vi "Read XML HW Configuration File_Parse Channels.vi"(8 "error in (no error)":errorcluster, 11 "channel1553":refnum<k24>[](array[refnum])) -> (0 "error out":errorcluster, 2 "channels":T1[](array[typedef]))   [LabVIEW 2017, in "Ballard 1553 System Explorer.lvlib"]
doc: "This VI parses the XML HW DB."
uses:
  Ballard 1553 System Explorer.lvlib
  Ballard_Channel.ctl
  Ballard_BC.ctl
  Ballard_message.ctl
  Ballard_messageType.ctl
  Ballard_CWD1.ctl
  Ballard_CWD2.ctl
  Ballard_minorFrame.ctl
  Ballard_majorFrame.ctl
  Ballard_acyclicFrame.ctl
  Ballard_RT.ctl
  Ballard_RT subAddress.ctl
  Ballard_RT direction.ctl
  Ballard_RT rtMode.ctl
  Ballard_RT modeCode.ctl
  D:/Ballard-1553-Custom-Device Inline Async/Source/System Explorer/SubVIs/Parse XML Ballard/Ballard_BTI_XML_MIL_STD_1553_Deserializer.dll
  Ballard_BTI_XML_MIL_STD_1553_Deserializer.dll
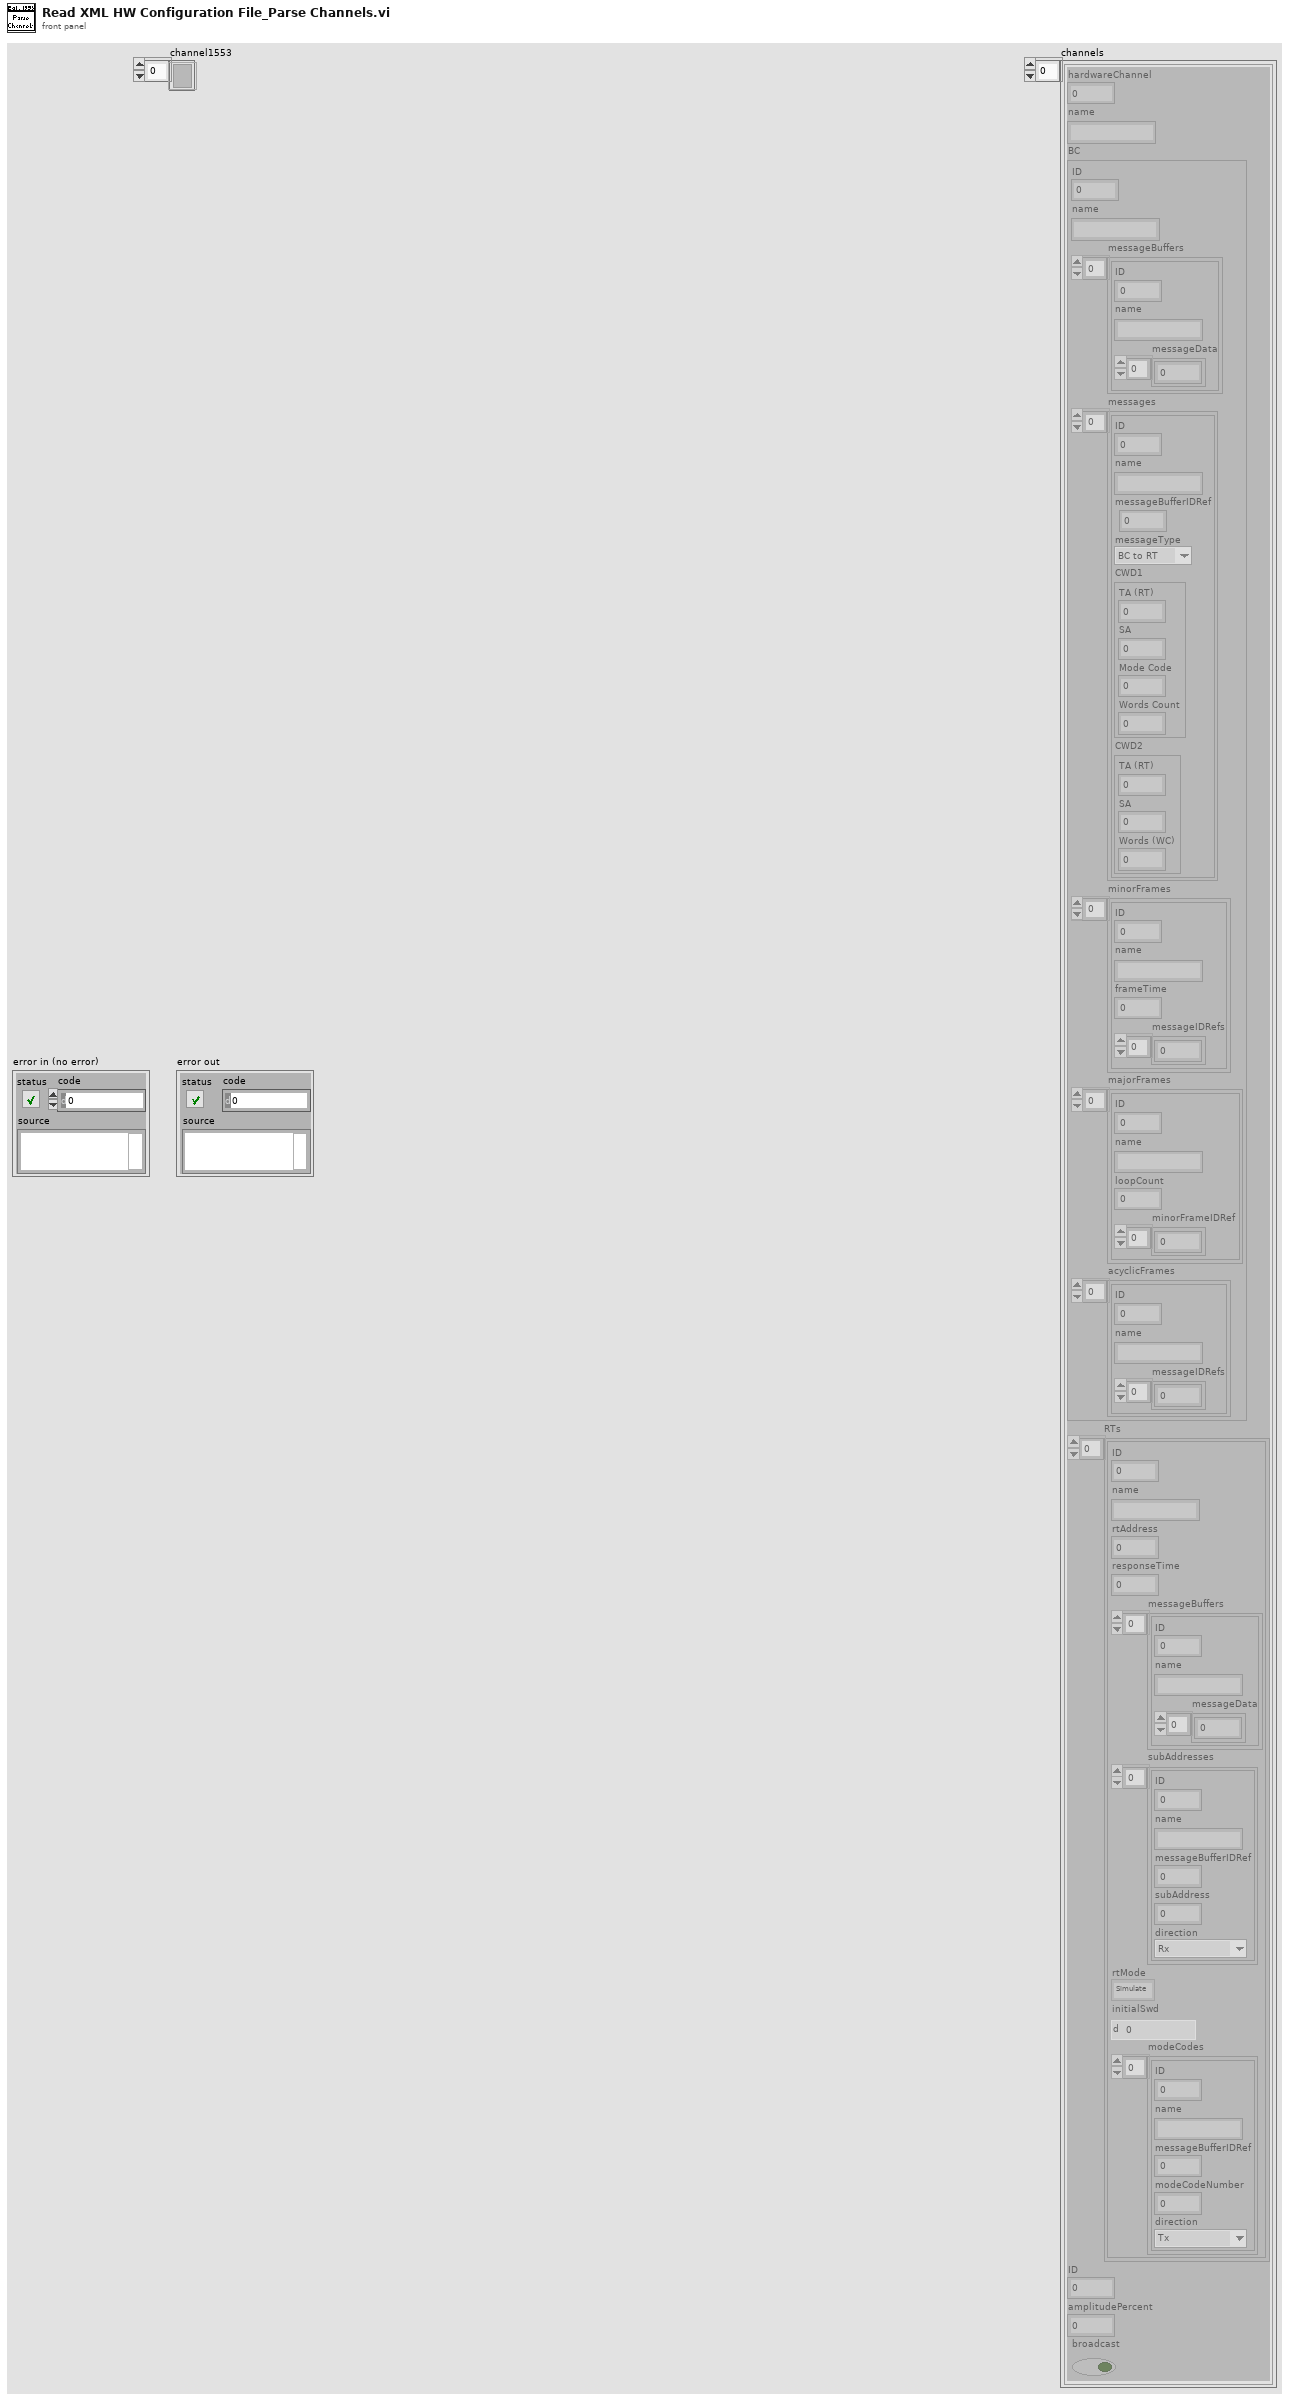
[diagram p1: front panel]
types:
  T1 = typedef "Ballard 1553 System Explorer.lvlib/Ballard_Channel.ctl" = cluster{"hardwareChannel":i32, "name":string, "BC":T2, "RTs":T10[], "ID":i32, "amplitudePercent":dbl, "broadcast":bool}
  T2 = typedef "Ballard 1553 System Explorer.lvlib/Ballard_BC.ctl" = cluster{"ID":i32, "name":string, "messageBuffers":cluster{"ID":i32, "name":string, "messageData":u16[]}[], "messages":T3[], "minorFrames":T7[], "majorFrames":T8[], "acyclicFrames":T9[]}
  T3 = typedef "Ballard 1553 System Explorer.lvlib/Ballard_message.ctl" = cluster{"ID":i32, "name":string, "messageBufferIDRef":i32, "messageType":T4, "CWD1":T5, "CWD2":T6}
  T4 = typedef "Ballard 1553 System Explorer.lvlib/Ballard_messageType.ctl" = enum16{"BC to RT", "RT to BC", "RT to RT", "MC (Rx)", "MC (Tx)"}
  T5 = typedef "Ballard 1553 System Explorer.lvlib/Ballard_CWD1.ctl" = cluster{"TA (RT)":i8, "SA":i8, "Mode Code":i8, "Words Count":i8}
  T6 = typedef "Ballard 1553 System Explorer.lvlib/Ballard_CWD2.ctl" = cluster{"TA (RT)":i8, "SA":i8, "Words (WC)":i8}
  T7 = typedef "Ballard 1553 System Explorer.lvlib/Ballard_minorFrame.ctl" = cluster{"ID":i32, "name":string, "frameTime":i32, "messageIDRefs":i32[]}
  T8 = typedef "Ballard 1553 System Explorer.lvlib/Ballard_majorFrame.ctl" = cluster{"ID":i32, "name":string, "loopCount":i32, "minorFrameIDRef":i32[]}
  T9 = typedef "Ballard 1553 System Explorer.lvlib/Ballard_acyclicFrame.ctl" = cluster{"ID":i32, "name":string, "messageIDRefs":i32[]}
  T10 = typedef "Ballard 1553 System Explorer.lvlib/Ballard_RT.ctl" = cluster{"ID":i32, "name":string, "rtAddress":i8, "responseTime":i32, "messageBuffers":cluster{"ID":i32, "name":string, "messageData":u16[]}[], "subAddresses":T11[], "rtMode":T13, "initialSwd":u16, "modeCodes":T14[]}
  T11 = typedef "Ballard 1553 System Explorer.lvlib/Ballard_RT subAddress.ctl" = cluster{"ID":i32, "name":string, "messageBufferIDRef":i32, "subAddress":i8, "direction":T12}
  T12 = typedef "Ballard 1553 System Explorer.lvlib/Ballard_RT direction.ctl" = enum16{"Tx", "Rx"}
  T13 = typedef "Ballard 1553 System Explorer.lvlib/Ballard_RT rtMode.ctl" = enum16{"Simulate", "Monitor", "Disable"}
  T14 = typedef "Ballard 1553 System Explorer.lvlib/Ballard_RT modeCode.ctl" = cluster{"ID":i32, "name":string, "messageBufferIDRef":i32, "modeCodeNumber":i8, "direction":T12}
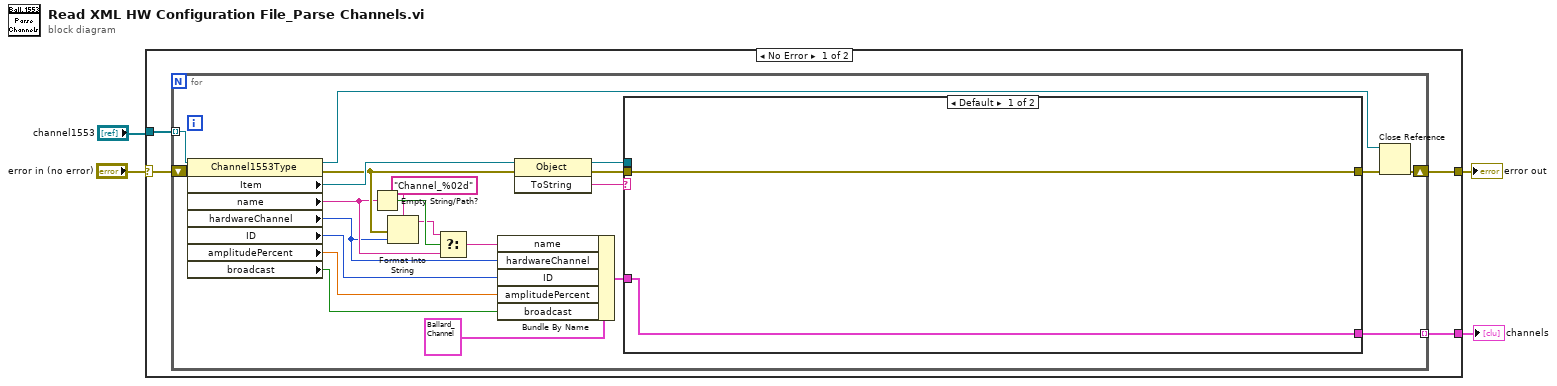
[diagram p0: block diagram]
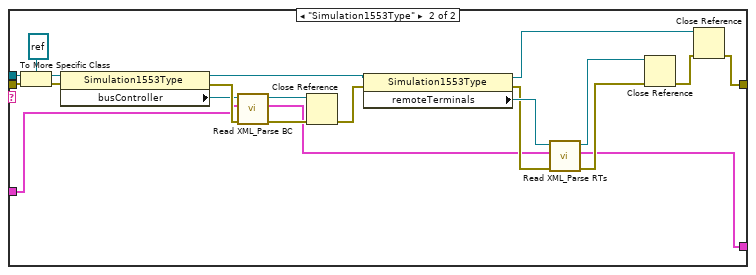
[diagram p2: hidden frame]
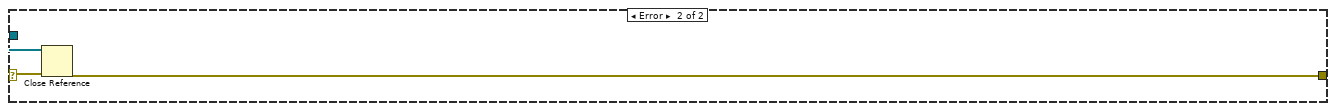
[diagram p3: hidden frame]
diagram:
  n1 = case shown="No Error" "error in (no error)" {
    selector: "error in (no error)" -> [w6 w55]
    tunnel: [w8 w54] -> w4
    tunnel: "channel1553" -> [w7 w56]
    tunnel: [w5 _] -> w2
    frame No Error {
      n2 = for {
        tunnel: w7 -> [w30] mode=indexing
        shift-right: [w23] -> w8
        shift-left: w6 -> [w27]
        tunnel: [w18] -> w5 mode=indexing
        n3 = property class="Channel1553Type"(reference=w30, error in=w27) -> (reference out=w22:refnum<k24>, error out=w15:errorcluster, "Item"=w25:refnum<k24>, "name"=w14:string, "hardwareChannel"=w10:i32, "ID"=w12:i32, "amplitudePercent"=w19:dbl, "broadcast"=w9:bool)
        n4 = Empty String/Path?(string/path=w14) -> (empty?=w17:bool)
        n5 = Format Into String(format string="Channel_%02d", error in=w15, w10) -> (resulting string=w16:string)  [unwired: 1 in, 1 out]
        n6 = Select(t=w16, s=w17, f=w14) -> (s? t:f=w11:string)
        n7 = Bundle By Name(cluster=T1 {"hardwareChannel"=0, "name"="", "BC"={"ID"=0, "name"="", "messageBuffers"=[], "messages"=[], "minorFrames"=[], "majorFrames"=[], "acyclicFrames"=[]}, "RTs"=[], "ID"=0, "amplitudePercent"=0.0, "broadcast"=FALSE} ("channel"), "name"=w11, "hardwareChannel"=w10, "ID"=w12, "amplitudePercent"=w19, "broadcast"=w9) -> (w20:T1)
        n8 = invoke class="Object" method="ToString"(reference=w25, error in=w15) -> (reference out=w28:refnum<k24>, error out=w26:errorcluster, "ToString"=w29:string)  [unwired: 1 in]
        n9 = case shown="Default" w29 {
          tunnel: w28 -> [_ w51]
          tunnel: w26 -> [w32 w52]
          tunnel: [w32 w47] -> w24
          tunnel: w20 -> [w31 w46]
          tunnel: [w31 w34] -> w18
          frame Default {
          }
          frame "Simulation1553Type" {
            n10 = To More Specific Class(target class=refnum<k24> refnum, reference=w51, error in=w52) -> (specific class reference=w50:refnum<k24>, error out=w49:errorcluster)
            n11 = property class="Simulation1553Type"(reference=w50, error in=w49) -> (reference out=w42:refnum<k24>, error out=w48:errorcluster, "busController"=w33:refnum<k24>)
            n12 = call "Read XML_Parse BC.vi"("error in (no error)"=w48, "channel"=w46, "BusController1553Type"=w33) -> ("error out"=w45:errorcluster, "channel out"=w35:T1, "BusController1553Type"=w44:refnum<k24>)  [unwired: 6 in]
            n13 = Close Reference(reference=w44, error in (no error)=w45) -> (error out=w43:errorcluster)
            n14 = property class="Simulation1553Type"(reference=w42, error in=w43) -> (reference out=w40:refnum<k24>, error out=w39:errorcluster, "remoteTerminals"=w41:refnum<k24>)
            n15 = call "Read XML_Parse RTs.vi"("error in (no error)"=w39, "channel in"=w35, "RemoteTerminals1553Type"=w41) -> ("error out"=w36:errorcluster, "channel out"=w34:T1, "RemoteTerminals1553Type"=w38:refnum<k24>)  [unwired: 6 in]
            n16 = Close Reference(reference=w38, error in (no error)=w36) -> (error out=w37:errorcluster)
            n17 = Close Reference(reference=w40, error in (no error)=w37) -> (error out=w47:errorcluster)
          }
        }
        n18 = Close Reference(reference=w22, error in (no error)=w24) -> (error out=w23:errorcluster)
      }
    }
    frame Error {
      n19 = Close Reference(reference=w56, error in (no error)=w55) -> (error out=w54:errorcluster)
    }
  }
  "error out" <- w4
  "channels" <- w2
